vi "dome_getSample_Summary.vi"(8 "error in (no error)":errorcluster, 11 "Summary_Ctl":T1={"example[16]"=[FALSE, FALSE, FALSE, FALSE, FALSE, FALSE, FALSE, FALSE, FALSE, FALSE, FALSE, FALSE, FALSE, FALSE, FALSE, FALSE]}) -> (0 "error out":errorcluster, 2 "function return":i32, 3 "Summary_Ctl out":T1)   [LabVIEW 2016, in "SALLV_dome.lvlib"]
doc: "int dome_shm_getSample_SummaryLV(dome_SummaryLV *Summary_Ctl );"
uses:
  SALLV_dome.lvlib
  DataTypes/Summary.ctl
  SALLV_dome.so
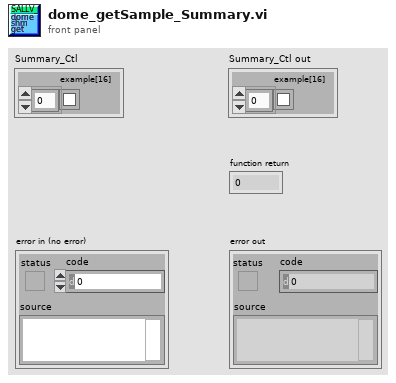
[diagram p1: front panel]
types:
  T1 = typedef "SALLV_dome.lvlib/Summary.ctl" = cluster{"example[16]":bool[]}
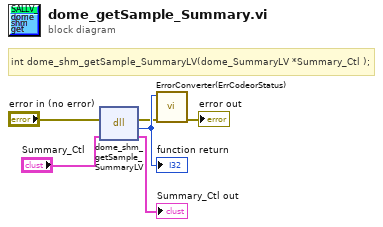
[diagram p0: block diagram]
diagram:
  # "int dome_shm_getSample_SummaryLV(dome_SummaryLV *Summary_Ctl );"
  n1 = dll-call lib="home/andres/Desktop/SALLV_dome/SALLV_dome.*" fn="dome_shm_getSample_SummaryLV"(error in="error in (no error)", "Summary_Ctl"="Summary_Ctl") -> (error out=w2:errorcluster, w6:i32, "Summary_Ctl"=→"Summary_Ctl out":T1)  [unwired: 2 in, 1 out]
  "function return" <- w6
  n2 = call "ErrorConverter(ErrCodeorStatus).vi"("error in (no error)"=w2, "error code"=w6) -> ("error out"=→"error out":errorcluster)  [unwired: 9 in]
